vi "log_event.vi"(6 "Message":string, 8 "error in":errorcluster, 9 "State":string, 10 "Facility":string, 11 "Severity":enum16{"OK", "Debug", "Warn", "Error"}(ring)) -> (0 "error out":errorcluster)   [LabVIEW 2013]
uses:
  log_event.ctl
panel:
  # "Send status event to logger.  See tip/description for documentation on arguments."
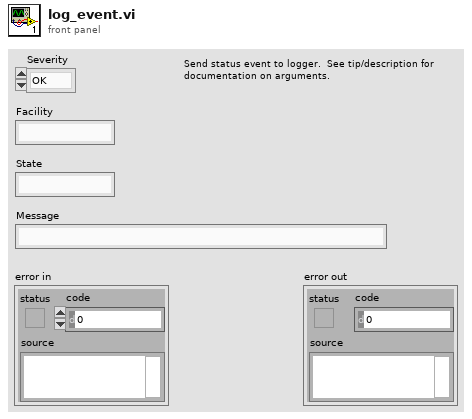
[diagram p1: front panel]
types:
  T1 = typedef "log_event.ctl" = cluster{"Facility ID":i32, "Severity":enum16{"OK", "Debug", "Warn", "Error"}, "Timestamp":timestamp, "Facility":string, "State":string, "Message":string}
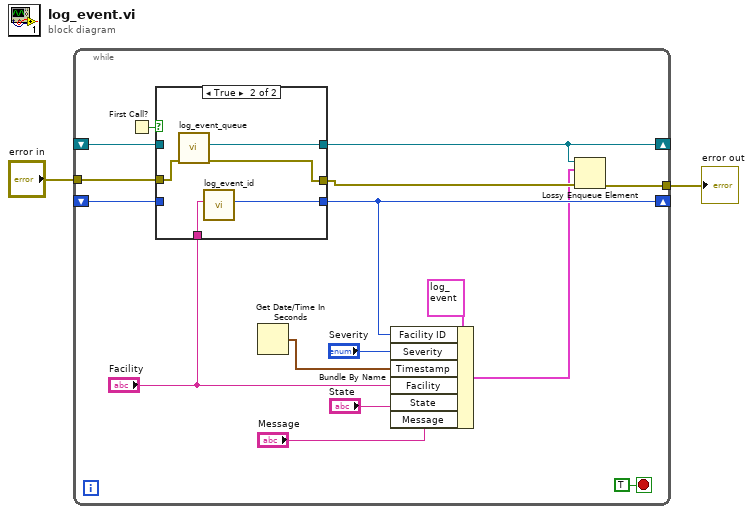
[diagram p0: block diagram]
diagram:
  n1 = while {
    shift-right: [w14] -> _
    shift-left: _ -> [w16]
    shift-right: [w10] -> _
    shift-left: _ -> [w15]
    tunnel: "error in" -> [w12]
    tunnel: [w5] -> w1
    stop <- TRUE stop-if-true
    n2 = First Call?() -> (First Call?: T/F=w17:bool)
    n3 = case shown="True" w17 {
      tunnel: [w21 w26] -> w14
      tunnel: w16 -> [w21 _]
      tunnel: [w20 w25] -> w10
      tunnel: w15 -> [w20 _]
      tunnel: w12 -> [w19 w24]
      tunnel: [w19 w23] -> w11
      tunnel: "Facility" -> [_ w22]
      frame False {
      }
      frame True {
        n4 = call "log_event_queue.vi"("error in"=w24) -> ("error out"=w23:errorcluster, "Log event queue"=w26:refnum<queue>)  [unwired: 9 in]
        n5 = call "log_event_id.vi"("Facility"=w22) -> ("Facility ID"=w25:i32)  [unwired: 10 in]
      }
    }
    n6 = Get Date/Time In Seconds() -> (seconds since 1Jan1904=w4:timestamp)
    n7 = Bundle By Name(cluster=T1 {"Facility ID"=0, "Severity"=enum."Debug", "Timestamp"=timestamp(0 s since 1904-01-01), "Facility"="", "State"="", "Message"=""} ("element"), "Facility ID"=w10, "Severity"="Severity", "Timestamp"=w4, "Facility"="Facility", "State"="State", "Message"="Message") -> (w6:T1)
    n8 = Lossy Enqueue Element(queue=w14, element=w6, error in (no error)=w11) -> (error out=w5:errorcluster)  [unwired: 3 out]
  }
  "error out" <- w1
